vi "Read Skipped Count.vi"(11 "Test Case Result In":refnum<class "Test Case Result.lvclass">) -> (2 "Skipped count":i32, 3 "Test Case Result Out":refnum<class "Test Case Result.lvclass">)   [LabVIEW 2020, in "Test Case Result.lvclass"]
uses:
  Test Case Result.lvclass
  Assertion Result/Public/TypeDefs/Status.ctl
  Test Case Result.lvclass/Test Case Result.ctl
  Method Result/Method Result.lvclass/Method Result.ctl
  Method Result/Public/Read Status.vi
  Assertion Result/Assertion Result.lvclass
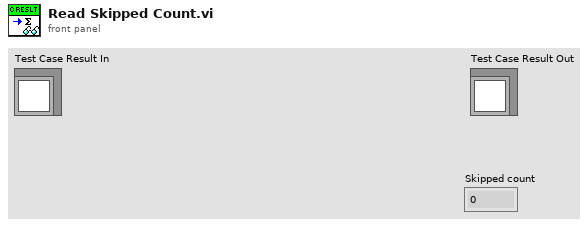
[diagram p1: front panel]
types:
  T1 = typedef "Assertion Result.lvclass/Status.ctl" = enum16{"Pass", "Fail", "Error", "Skipped", "Setup Error", "Broken", "Teardown Error"}
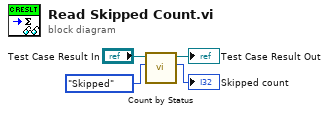
[diagram p0: block diagram]
diagram:
  n1 = call "Count by Status.vi"("Status"=Status."Skipped", "Test Case Result In"="Test Case Result In") -> ("Count"=→"Skipped count":i32, "Test Case Result Out"=→"Test Case Result Out":refnum<class "Test Case Result.lvclass">)  [unwired: 8 in]
